vi "Understanding Loops.vi"() -> ()   [LabVIEW 2026]
panel:
  in  "stop":bool
  out "Celsius Indicator":dbl
  out "Fahrenheit Indicator":dbl
  in  "Celsius":dbl(slide) scale=0.0..100.0
  out "Fahrenheit":dbl(slide) scale=0.0..500.0
  # "Understanding Loops"
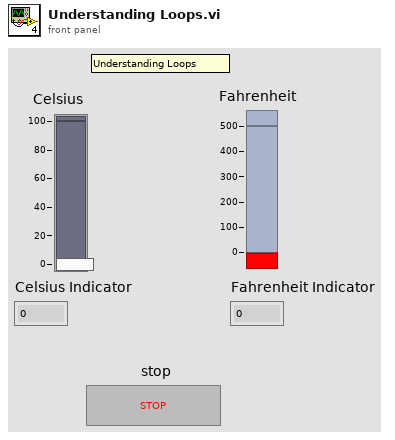
[diagram p1: front panel]
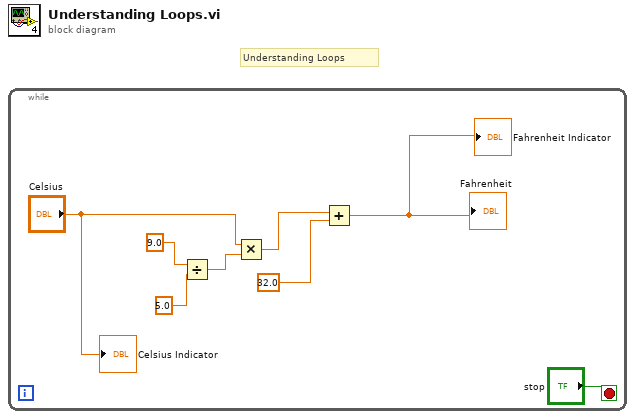
[diagram p0: block diagram]
diagram:
  # "Understanding Loops"
  n1 = while {
    stop <- "stop" stop-if-true
    n2 = Divide(x=9.0, y=5.0) -> (x/y=w7:dbl)
    n3 = Multiply(x="Celsius", y=w7) -> (x*y=w6:dbl)
    n4 = Add(x=w6, y=32.0) -> (x+y=→"Fahrenheit" →"Fahrenheit Indicator":dbl)
    "Celsius Indicator" <- "Celsius"
  }
